vi "Get VI FP Data.vi"(8 "error in (no error)":errorcluster, 11 "VI ref in":refnum<vi>) -> (0 "error out":errorcluster, 2 "FP Data":T1, 3 "VI ref out":refnum<vi>)   [LabVIEW 2019]
uses:
  <vilib>/Utility/miscctls.llb/LVPositionTypeDef.ctl
  <vilib>/Utility/miscctls.llb/LVBoundsTypeDef.ctl
  Typedefs/FP Data.ctl
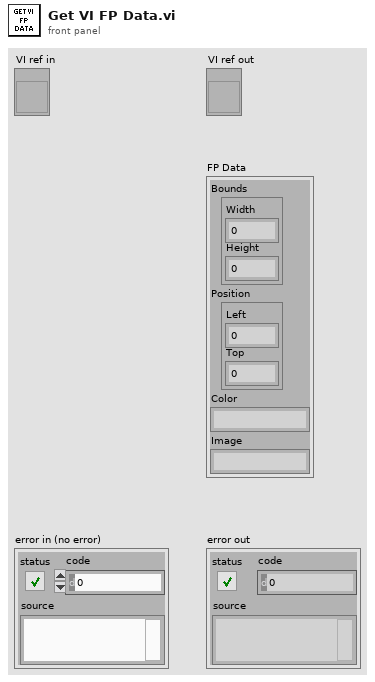
[diagram p1: front panel]
types:
  T1 = typedef "FP Data.ctl" = cluster{"Bounds":T2, "Position":T3, "Color":string, "Image":string}
  T2 = typedef "LVBoundsTypeDef.ctl" = cluster{"Width":u32, "Height":u32}
  T3 = typedef "LVPositionTypeDef.ctl" = cluster{"Left":i32, "Top":i32}
  T4 = typedef "imagedata.ctl" = cluster{"image type":i32, "image depth":i32, "image":u8[], "mask":u8[], "colors":u32[], "Rectangle":cluster{"left":i16, "top":i16, "right":i16, "bottom":i16}}
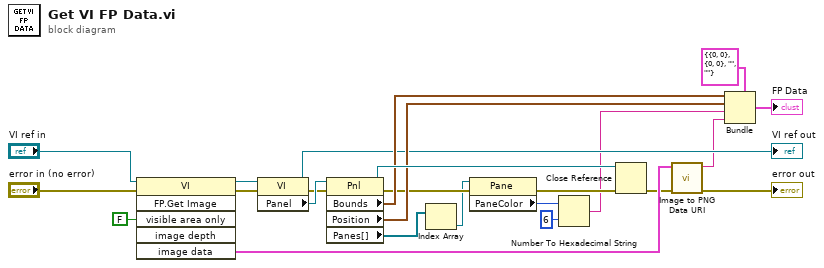
[diagram p0: block diagram]
diagram:
  n1 = invoke class="VI" method="FP.Get Image"(reference="VI ref in", error in="error in (no error)", "visible area only"=FALSE ("Visible Area Only")) -> (reference out=w22:refnum<vi>, error out=w21:errorcluster, "image data"=w15:T4)  [unwired: 3 in, 3 out]
  n2 = property class="VI"(reference=w22, error in=w21) -> (reference out=→"VI ref out":refnum<vi>, error out=w23:errorcluster, "Panel"=w24:refnum<vi>)
  n3 = property class="Pnl"(reference=w24, error in=w23) -> (reference out=w20:refnum<vi>, error out=w11:errorcluster, "Bounds"=w19:T2, "Position"=w18:T3, "Panes[]"=w12:refnum<vi>[])
  n4 = Index Array(array=w12) -> (element=w9:refnum<vi>)  [unwired: 1 in]
  n5 = property class="Pane"(reference=w9, error in=w11) -> (error out=w10:errorcluster, "PaneColor"=w7:u32)  [unwired: 1 out]
  n6 = Number To Hexadecimal String(1:i16 6 ("width (-)"), 2:w7) -> (0:w5:string)
  n7 = Close Reference(reference=w20, error in (no error)=w10) -> (error out=w13:errorcluster)
  n8 = call "Image to PNG Data URI.vi"("error in (no error)"=w13, "Image data"=w15) -> ("error out"=→"error out":errorcluster, "Base64 encoded"=w6:string)  [unwired: 7 in, 1 out]
  n9 = Bundle(cluster=T1 {"Bounds"={"Width"=0, "Height"=0}, "Position"={"Left"=0, "Top"=0}, "Color"="", "Image"=""} ("FP"), "Bounds"=w19, "Position"=w18, "Color"=w5, "Image"=w6) -> (→"FP Data":T1)
